vi "Image2WallDistances.vi"(3 "error in (no error)":errorcluster, 5 "Image Src":T1) -> (0 "error out":errorcluster)   [LabVIEW 2009, in "ImageAnalysis.lvlib"]
uses:
  ImageAnalysis.lvlib
  <vilib>/vision/Image Controls.llb/IMAQ Image.ctl
  ImageProcessing.lvlib
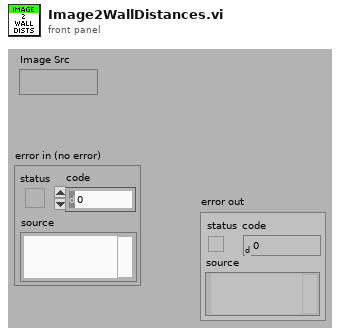
[diagram p1: front panel]
types:
  T1 = typedef "IMAQ Image.ctl" = refnum<image>
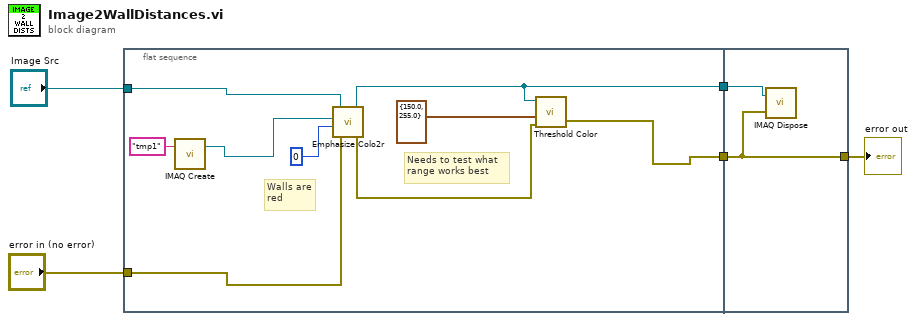
[diagram p0: block diagram]
diagram:
  n1 = flat-sequence {
    tunnel: "Image Src" -> [w9]
    tunnel: "error in (no error)" -> [w8]
    tunnel: [w7] -> w3
    tunnel: [w6] -> w1
    tunnel: w3 -> [w16]
    tunnel: [w16] -> w2
    tunnel: w1 -> [w15]
    frame #0 {
      # "Needs to test what \nrange works best"
      # "Walls are\nred"
      n2 = call "IMAQ Create"("Image Name"="tmp1") -> ("New Image"=w10:T1)  [unwired: 4 in, 1 out]
      n3 = call "Emphasize Colo2r.vi"("error in (no error)"=w8, "Color"=i8 0, "Image Dst"=w10, "Image Src"=w9) -> ("error out"=w14:errorcluster, "Image Out"=w6:T1)
      n4 = call "Threshold Color.vi"("error in (no error)"=w14, "Range"=cluster{"Lower value":sgl, "Upper value":sgl} {"Lower value"=150.0, "Upper value"=255.0}, "Image Src"=w6) -> ("error out"=w7:errorcluster)  [unwired: 1 in, 1 out]
    }
    frame #1 {
      n5 = call "IMAQ Dispose"("Image"=w15, "error in (no error)"=w16) -> ()  [unwired: 4 in, 1 out]
    }
  }
  "error out" <- w2
